vi "_divide float.vi"(6 "label":T1, 8 "i":errorcluster, 10 "B":T2, 11 "A":refnum<class "Value.lvclass">) -> (0 "error out":errorcluster, 2 "c":refnum<class "Value.lvclass">, 3 "A out":refnum<class "Value.lvclass">)   [LabVIEW 2023, in "LabGRAD.lvlib" / "Value.lvclass"]
uses:
  Value.lvclass
  Value.lvclass/Value.ctl
  UiObjects/numeric value control.ctl
  UiObjects/UiObjects.lvclass
  UiObjects/string control.ctl
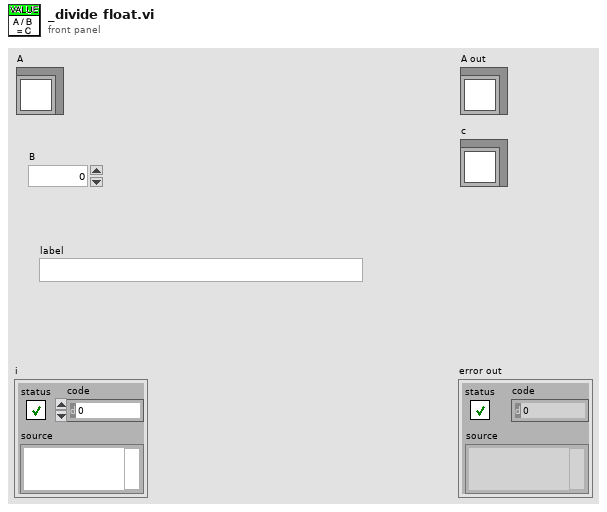
[diagram p1: front panel]
types:
  T1 = typedef "UiObjects.lvlib/UiObjects.lvclass/string control.ctl" = string
  T2 = typedef "UiObjects.lvlib/UiObjects.lvclass/numeric value control.ctl" = dbl
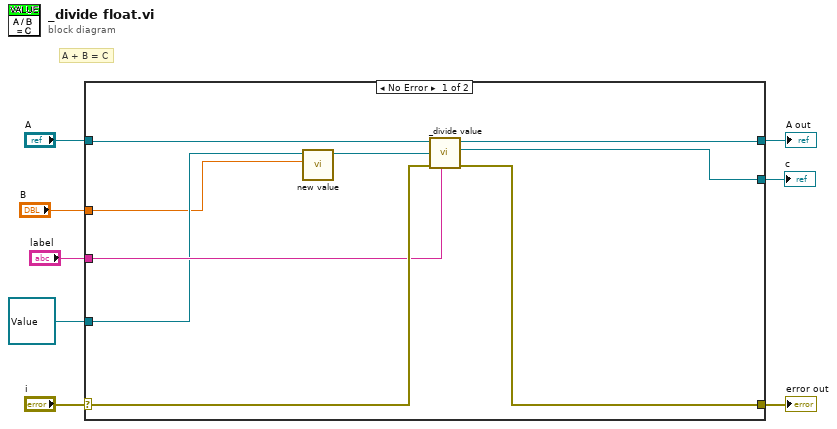
[diagram p0: block diagram]
diagram:
  # "A + B = C"
  n1 = case shown="No Error" "i" {
    selector: "i" -> [w14 w20]
    tunnel: [w13 w20] -> w7
    tunnel: [w16 w19] -> w5
    tunnel: "A" -> [w17 w19]
    tunnel: [w15 w18] -> w4
    tunnel: refnum<class "Value.lvclass"> refnum ("B") -> [w10 w18]
    tunnel: "B" -> [w9 _]
    tunnel: "label" -> [w12 _]
    frame No Error {
      n2 = call "new value.vi"("data"=w9, "Value in"=w10) -> ("Value out"=w11:refnum<class "Value.lvclass">)  [unwired: 8 in, 1 out]
      n3 = call "_divide value.vi"("label"=w12, "error in (no error)"=w14, "B"=w11, "A"=w17) -> ("error out"=w13:errorcluster, "C"=w15:refnum<class "Value.lvclass">, "A out"=w16:refnum<class "Value.lvclass">)  [unwired: 5 in]
    }
    frame Error {
    }
  }
  "error out" <- w7
  "A out" <- w5
  "c" <- w4
